vi "LVIS_CrcCalc.vi"(0 "String IN":string) -> (4 "CRC":string)   [LabVIEW 2015]
doc: "Calculates the event data CRC value."
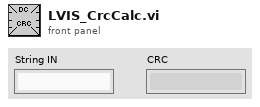
[diagram p1: front panel]
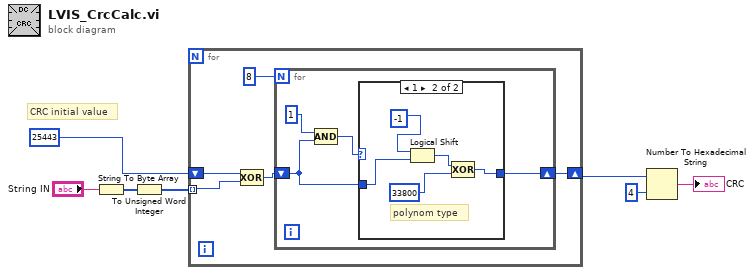
[diagram p0: block diagram]
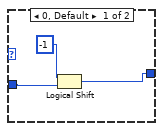
[diagram p2: hidden frame]
diagram:
  # "CRC initial value"
  n1 = String To Byte Array(string="String IN") -> (unsigned byte array=w6:u8[])
  n2 = To Unsigned Word Integer(number=w6) -> (unsigned 16bit integer=w5:u16[])
  n3 = for {
    shift-right: [w9] -> w4
    shift-left: u16 25443 -> [w10]
    tunnel: w5 -> [w8] mode=indexing
    n4 = Compound Arithmetic op=XOR(w10, w8) -> (w11:u32)
    n5 = for {
      N: 8 -> [_]
      shift-right: [w15] -> w9
      shift-left: w11 -> [w14]
      n6 = Compound Arithmetic op=AND(u16 1, w14) -> (w13:u32)
      n7 = case shown="1" w13 {
        tunnel: [w18 w23] -> w15
        tunnel: w14 -> [w17 w20]
        frame 0, Default {
          n8 = Logical Shift(y=i16 -1, x=w17) -> (x << y=w18:u32)
        }
        frame 1 {
          # "polynom type"
          n9 = Logical Shift(y=i16 -1, x=w20) -> (x << y=w22:u32)
          n10 = Compound Arithmetic op=XOR(w22, u32 33800) -> (w23:u32)
        }
      }
    }
  }
  n11 = Number To Hexadecimal String(1:i16 4 ("width (-)"), 2:w4) -> (0:→"CRC":string)
